vi "AUTON_Index.vi"(0 "Auton Array":dbl[][](array[numeric]), 5 "MeasuredHeading":dbl, 7 "LeftEncoder":dbl, 9 "RightEncoder":dbl) -> (4 "Right Drive":dbl, 6 "Left Drive":dbl, 8 "Harvester":dbl, 10 "Winch":dbl, 14 "Roller":dbl, 15 "Cam":dbl)   [LabVIEW 2013]
uses:
  Robot Global Data.vi
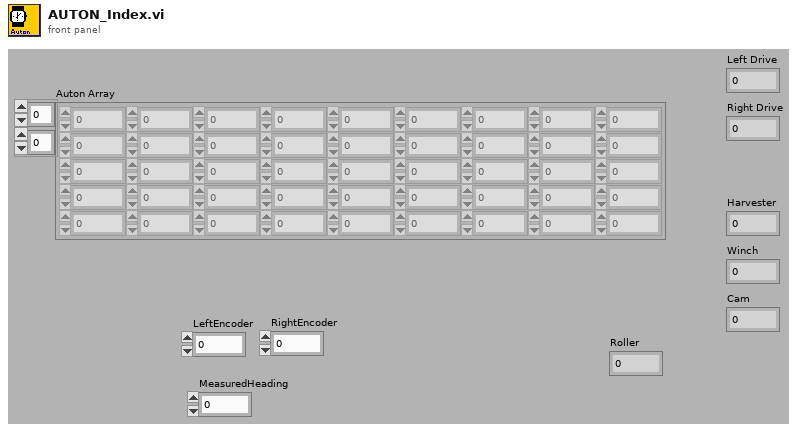
[diagram p1: front panel]
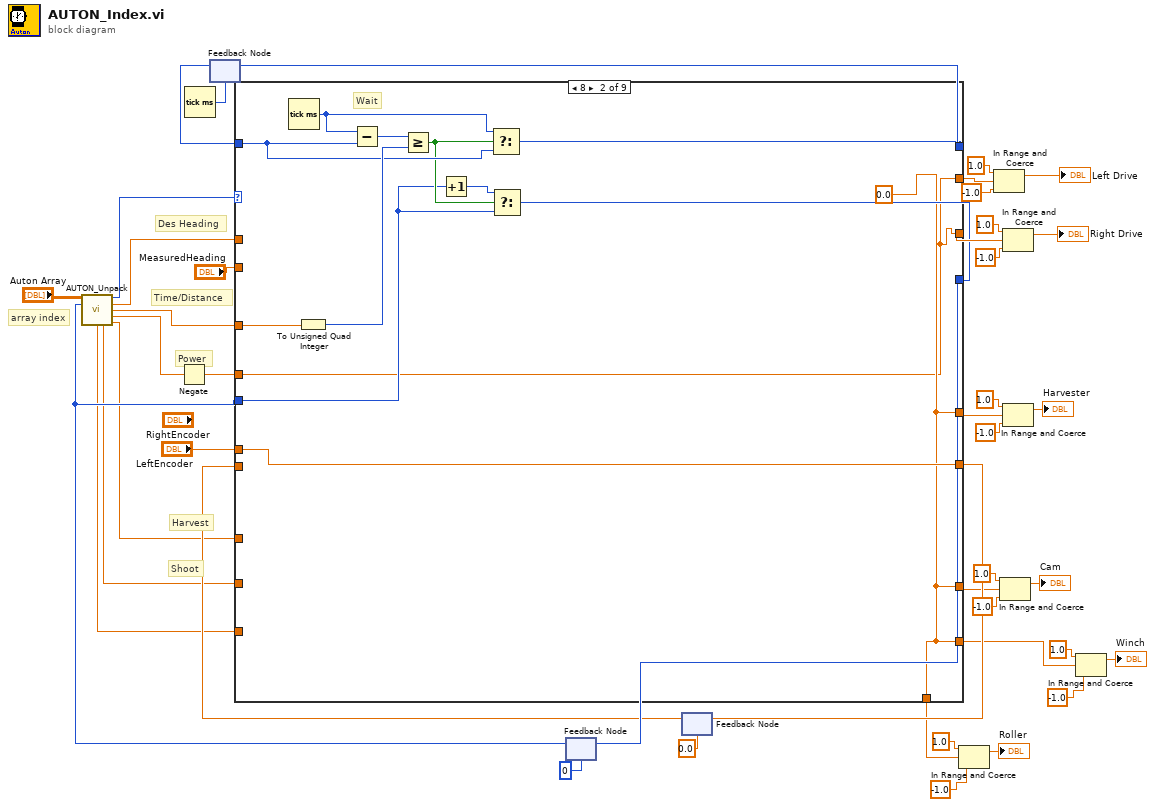
[diagram p0: block diagram]
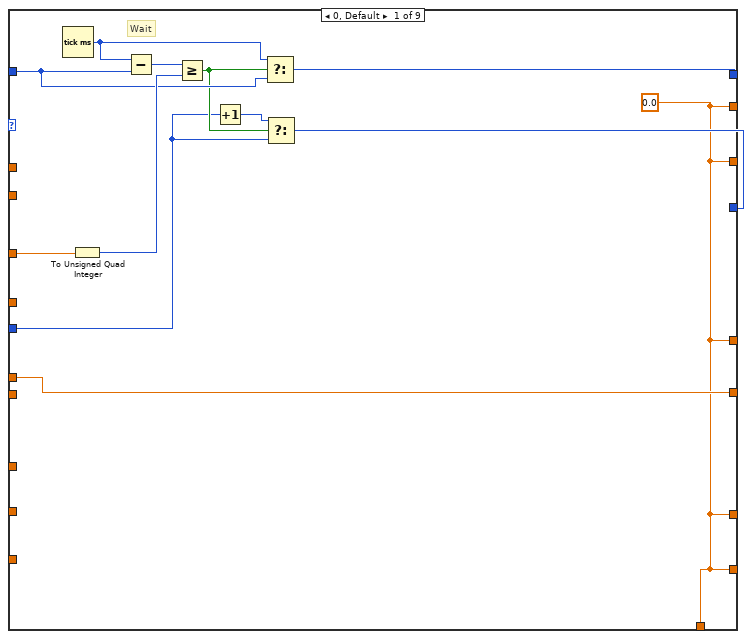
[diagram p2: hidden frame]
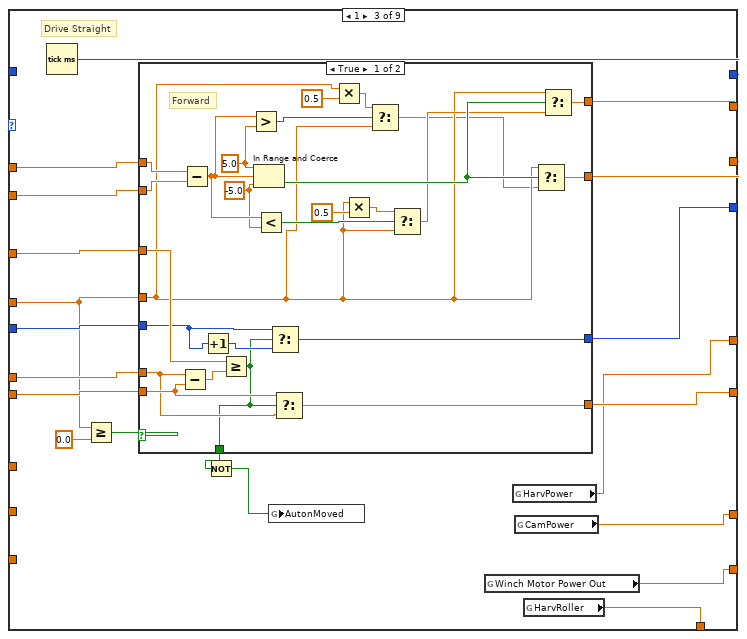
[diagram p3: hidden frame]
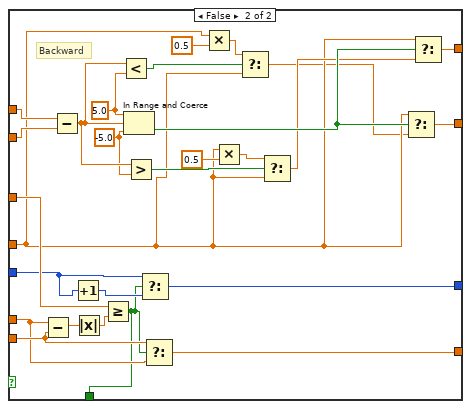
[diagram p4: hidden frame]
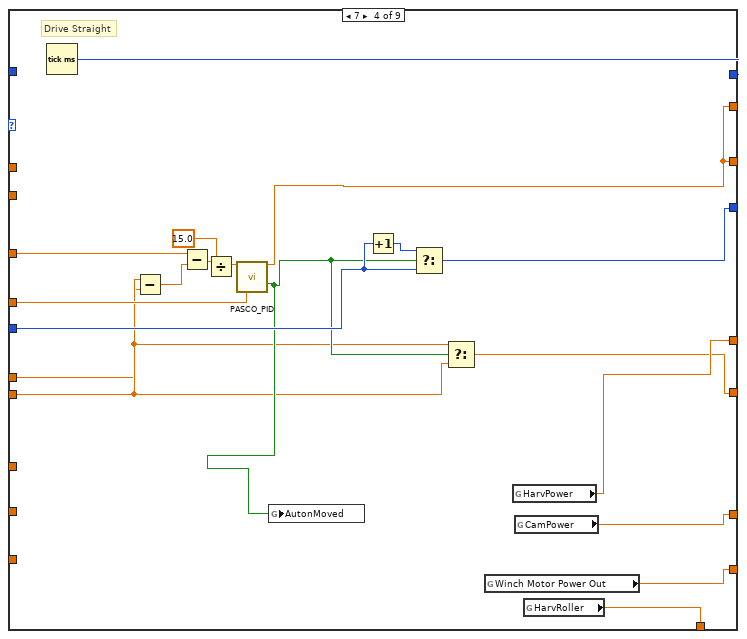
[diagram p5: hidden frame]
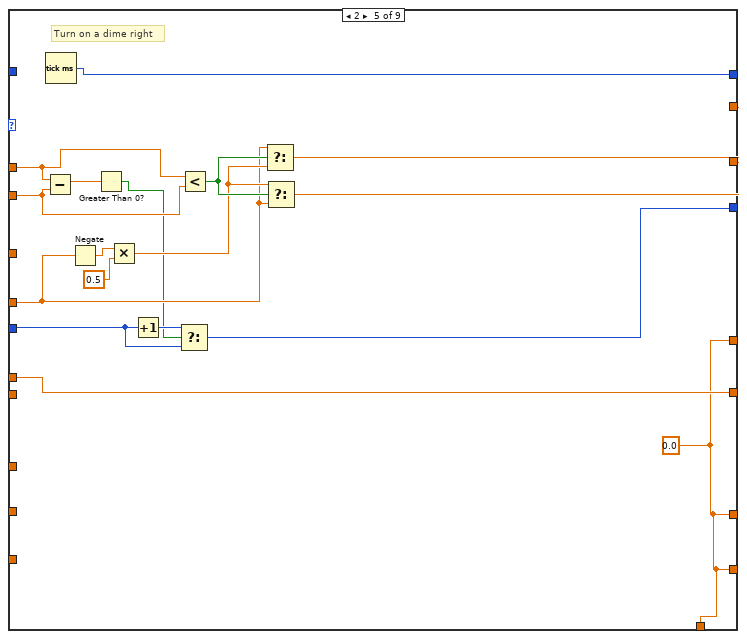
[diagram p6: hidden frame]
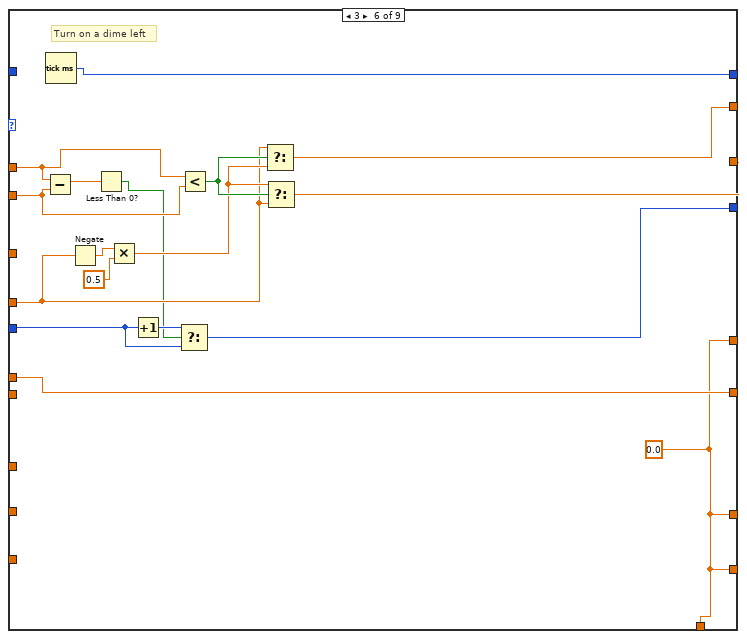
[diagram p7: hidden frame]
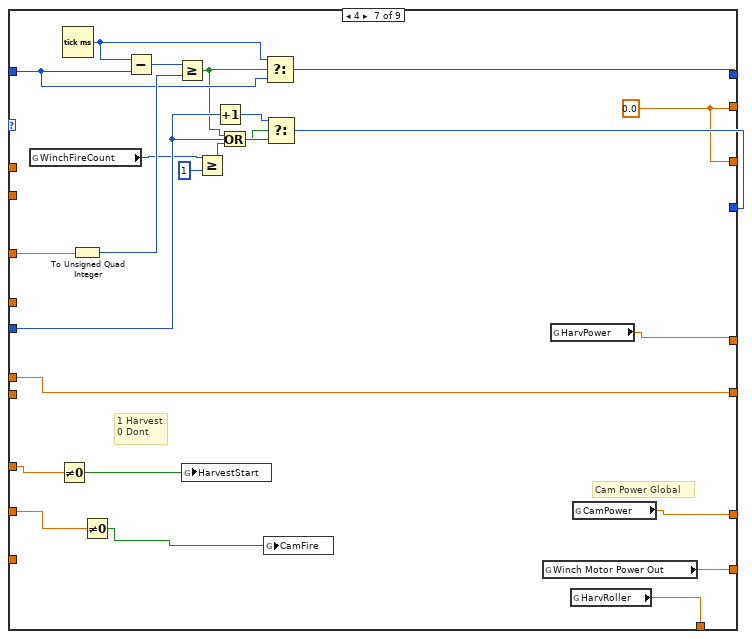
[diagram p8: hidden frame]
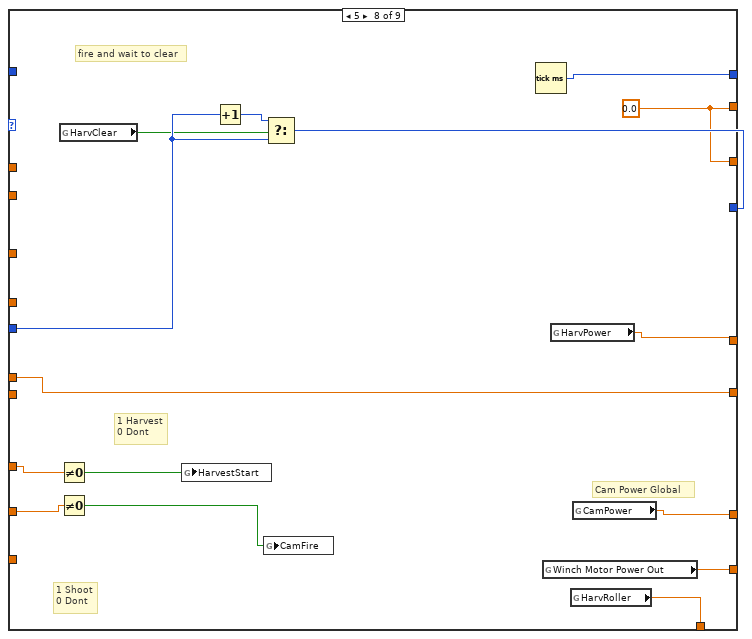
[diagram p9: hidden frame]
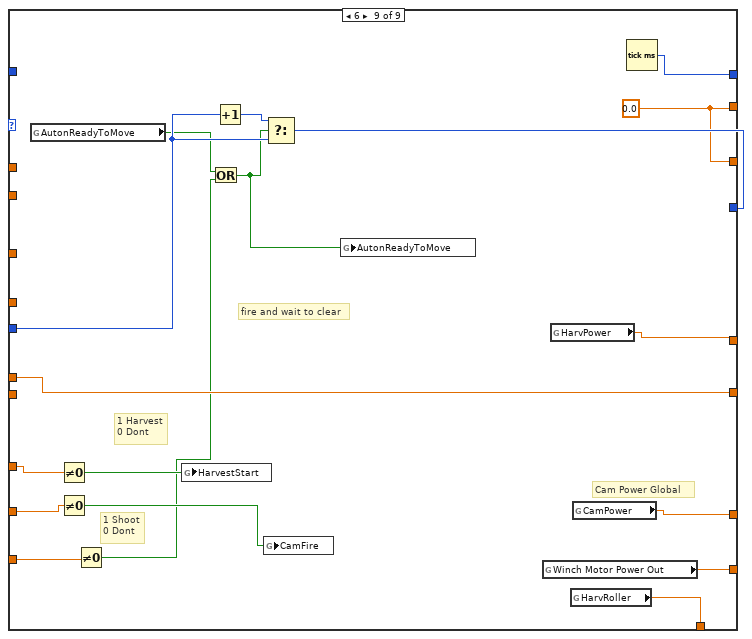
[diagram p10: hidden frame]
diagram:
  # "Shoot"
  # "Harvest"
  # "Des Heading"
  # "Time/Distance"
  # "Power"
  # "array index"
  n1 = Tick Count (ms)() -> (millisecond timer value=w42:u32)
  n2 = feedback #1(w42) -> (w43:u32)
  n3 = feedback #2(0) -> (w23:i32)
  n4 = call "AUTON_Unpack.vi"("all rows"="Auton Array", "Index"=w23) -> ("Primitive ID"=w26:i16, "Desired Heading"=w25:dbl, "Time/Distance"=w24:dbl, "Power"=w11:dbl, "Moved"=w1:dbl, "Shoot"=w8:dbl, "Harvest"=w9:dbl)  [unwired: 7 in]
  n5 = Negate(x=w11) -> (-x=w10:dbl)
  n6 = feedback #3(0.0) -> (w28:dbl)
  n7 = case shown="8" w26 {
    tunnel: [w48 w61 w87 w155 w173 w190 w212 w232 w250] -> w30
    tunnel: w23 -> [w49 w62 w82 w153 w176 w193 w213 w233 w251]
    tunnel: [w56 w69 w79 w161 w178 w195 w219 w223 w239] -> w32
    tunnel: w43 -> [w53 w66 _ _ _ _ w216 _ _]
    tunnel: w24 -> [w47 w60 w88 w145 _ _ w211 _ _]
    tunnel: w25 -> [_ _ w86 _ w171 w188 _ _ _]
    tunnel: [w45 w57 w84 w143 w174 w191 w210 w231 w249] -> w40
    tunnel: [w45 w57 w83 w143 w175 w192 w210 w231 w249] -> w33
    tunnel: w10 -> [_ w57 w78 w156 w165 w182 _ _ _]
    tunnel: "LeftEncoder" -> [w46 w59 w80 w148 w172 w189 w209 w230 w248]
    tunnel: "MeasuredHeading" -> [_ _ w85 _ w170 w187 _ _ _]
    tunnel: w28 -> [_ _ w81 w149 _ _ _ _ _]
    tunnel: [w46 w59 w89 w151 w172 w189 w209 w230 w248] -> w27
    tunnel: [w45 w58 w75 w160 w162 w179 w207 w228 w246] -> w13
    tunnel: [w45 w58 w73 w158 w162 w179 w208 w229 w247] -> w12
    tunnel: w9 -> [_ _ _ _ _ _ w204 w226 w244]
    tunnel: w8 -> [_ _ _ _ _ _ w206 w221 w241]
    tunnel: [w45 w58 w74 w159 w162 w179 w205 w227 w245] -> w7
    tunnel: [w45 w58 w72 w157 w162 w179 w201 w224 w242] -> w3
    tunnel: w1 -> [_ _ _ _ _ _ _ _ w238]
    frame 0, Default {
      w45 = 0.0 ("Numeric")
      # "Wait"
      n8 = Tick Count (ms)() -> (millisecond timer value=w52:u32)
      n9 = To Unsigned Quad Integer(1:w47) -> (0:w54:u64)
      n10 = Subtract(x=w52, y=w53) -> (x-y=w55:u32)
      n11 = Greater Or Equal?(x=w55, y=w54) -> (x >= y?=w51:bool)
      n12 = Increment(x=w49) -> (x+1=w50:i32)
      n13 = Select(t=w52, s=w51, f=w53) -> (s? t:f=w56:u32)
      n14 = Select(t=w50, s=w51, f=w49) -> (s? t:f=w48:i32)
    }
    frame 8 {
      w58 = 0.0 ("Numeric")
      # "Wait"
      n15 = Tick Count (ms)() -> (millisecond timer value=w65:u32)
      n16 = To Unsigned Quad Integer(1:w60) -> (0:w67:u64)
      n17 = Subtract(x=w65, y=w66) -> (x-y=w68:u32)
      n18 = Greater Or Equal?(x=w68, y=w67) -> (x >= y?=w64:bool)
      n19 = Increment(x=w62) -> (x+1=w63:i32)
      n20 = Select(t=w65, s=w64, f=w66) -> (s? t:f=w69:u32)
      n21 = Select(t=w63, s=w64, f=w62) -> (s? t:f=w61:i32)
    }
    frame 1 {
      # "Drive Straight"
      n22 = Tick Count (ms)() -> (millisecond timer value=w79:u32)
      n23 = Greater Or Equal?(x=w78, y=0.0) -> (x >= y?=w76:bool)
      n24 = case shown="True" w76 {
        tunnel: [w115 w142] -> w89
        tunnel: w88 -> [w113 w141]
        tunnel: [w112 w140] -> w87
        tunnel: w86 -> [w111 w139]
        tunnel: w85 -> [w110 w138]
        tunnel: [w108 w136] -> w84
        tunnel: [w107 w135] -> w83
        tunnel: w78 -> [w96 w124]
        tunnel: w82 -> [w93 w121]
        tunnel: w81 -> [w92 w120]
        tunnel: w80 -> [w91 w119]
        tunnel: [w90 w116] -> w71
        frame True {
          w104 = -5.0 ("lower limit")
          w106 = 5.0 ("upper limit")
          # "Forward"
          n25 = Subtract(x=w91, y=w92) -> (x-y=w114:dbl)
          n26 = Subtract(x=w111, y=w110) -> (x-y=w105:dbl)
          n27 = Increment(x=w93) -> (x+1=w94:i32)
          n28 = Greater Or Equal?(x=w113, y=w114) -> (x >= y?=w90:bool)
          n29 = Greater?(x=w105, y=w106) -> (0:w99:bool)
          n30 = In Range and Coerce(upper limit=w106, x=w105, lower limit=w104) -> (In Range?=w109:bool)  [unwired: 1 out]
          n31 = Less?(x=w105, y=w104) -> (x < y?=w103:bool)
          n32 = Select(t=w93, s=w90, f=w94) -> (s? t:f=w112:i32)
          n33 = Select(t=w92, s=w90, f=w91) -> (s? t:f=w115:dbl)
          n34 = Multiply(x=w96, y=0.5) -> (x*y=w98:dbl)
          n35 = Multiply(x=w96, y=0.5) -> (x*y=w101:dbl)
          n36 = Select(t=w98, s=w99, f=w96) -> (s? t:f=w95:dbl)
          n37 = Select(t=w101, s=w103, f=w96) -> (s? t:f=w100:dbl)
          n38 = Select(t=w96, s=w109, f=w95) -> (s? t:f=w107:dbl)
          n39 = Select(t=w96, s=w109, f=w100) -> (s? t:f=w108:dbl)
        }
        frame False {
          w132 = -5.0 ("lower limit")
          w134 = 5.0 ("upper limit")
          # "Backward"
          n40 = Subtract(x=w119, y=w120) -> (x-y=w117:dbl)
          n41 = Subtract(x=w139, y=w138) -> (x-y=w133:dbl)
          n42 = Increment(x=w121) -> (x+1=w122:i32)
          n43 = Absolute Value(x=w117) -> (abs(x)=w118:dbl)
          n44 = Greater Or Equal?(x=w141, y=w118) -> (x >= y?=w116:bool)
          n45 = Less?(x=w133, y=w134) -> (x < y?=w127:bool)
          n46 = In Range and Coerce(upper limit=w134, x=w133, lower limit=w132) -> (In Range?=w137:bool)  [unwired: 1 out]
          n47 = Greater?(x=w133, y=w132) -> (0:w131:bool)
          n48 = Select(t=w121, s=w116, f=w122) -> (s? t:f=w140:i32)
          n49 = Select(t=w120, s=w116, f=w119) -> (s? t:f=w142:dbl)
          n50 = Multiply(x=w124, y=0.5) -> (x*y=w126:dbl)
          n51 = Multiply(x=w124, y=0.5) -> (x*y=w129:dbl)
          n52 = Select(t=w126, s=w127, f=w124) -> (s? t:f=w123:dbl)
          n53 = Select(t=w129, s=w131, f=w124) -> (s? t:f=w128:dbl)
          n54 = Select(t=w124, s=w137, f=w123) -> (s? t:f=w135:dbl)
          n55 = Select(t=w124, s=w137, f=w128) -> (s? t:f=w136:dbl)
        }
      }
      n56 = Not(x=w71) -> (.not. x?=w70:bool)
      n57 = global write "Robot Global Data.vi" "AutonMoved"(w70) -> ()
      n58 = global read "Robot Global Data.vi" "Winch Motor Power Out"() -> (w74:dbl)
      n59 = global read "Robot Global Data.vi" "HarvPower"() -> (w73:dbl)
      n60 = global read "Robot Global Data.vi" "CamPower"() -> (w75:dbl)
      n61 = global read "Robot Global Data.vi" "HarvRoller"() -> (w72:dbl)
    }
    frame 7 {
      # "Drive Straight"
      n62 = Tick Count (ms)() -> (millisecond timer value=w161:u32)
      n63 = Subtract(x=w149, y=w148) -> (x-y=w150:dbl)
      n64 = Subtract(x=w145, y=w150) -> (x-y=w146:dbl)
      n65 = Divide(x=w146, y=15.0) -> (x/y=w147:dbl)
      n66 = call "PASCO_PID.vi"("Delta"=w147, "P Gain"=w156) -> ("Output"=w143:dbl, "IsThere"=w152:bool)  [unwired: 12 in]
      n67 = global write "Robot Global Data.vi" "AutonMoved"(w152) -> ()
      n68 = Increment(x=w153) -> (x+1=w154:i32)
      n69 = Select(t=w154, s=w152, f=w153) -> (s? t:f=w155:i32)
      n70 = Select(t=w148, s=w152, f=w149) -> (s? t:f=w151:dbl)
      n71 = global read "Robot Global Data.vi" "Winch Motor Power Out"() -> (w159:dbl)
      n72 = global read "Robot Global Data.vi" "HarvPower"() -> (w158:dbl)
      n73 = global read "Robot Global Data.vi" "CamPower"() -> (w160:dbl)
      n74 = global read "Robot Global Data.vi" "HarvRoller"() -> (w157:dbl)
    }
    frame 2 {
      w162 = 0.0 ("Numeric")
      # "Turn on a dime right"
      n75 = Subtract(x=w171, y=w170) -> (x-y=w164:dbl)
      n76 = Tick Count (ms)() -> (millisecond timer value=w178:u32)
      n77 = Negate(x=w165) -> (-x=w168:dbl)
      n78 = Greater Than 0?(x=w164) -> (x > 0?=w163:bool)
      n79 = Multiply(x=w168, y=0.5) -> (x*y=w166:dbl)
      n80 = Increment(x=w176) -> (x+1=w177:i32)
      n81 = Select(t=w177, s=w163, f=w176) -> (s? t:f=w173:i32)
      n82 = Less?(x=w171, y=w170) -> (x < y?=w169:bool)
      n83 = Select(t=w165, s=w169, f=w166) -> (s? t:f=w174:dbl)
      n84 = Select(t=w166, s=w169, f=w165) -> (s? t:f=w175:dbl)
    }
    frame 3 {
      w179 = 0.0 ("Numeric")
      # "Turn on a dime left"
      n85 = Subtract(x=w188, y=w187) -> (x-y=w181:dbl)
      n86 = Tick Count (ms)() -> (millisecond timer value=w195:u32)
      n87 = Negate(x=w182) -> (-x=w185:dbl)
      n88 = Less Than 0?(x=w181) -> (x < 0?=w180:bool)
      n89 = Multiply(x=w185, y=0.5) -> (x*y=w183:dbl)
      n90 = Increment(x=w193) -> (x+1=w194:i32)
      n91 = Select(t=w194, s=w180, f=w193) -> (s? t:f=w190:i32)
      n92 = Less?(x=w188, y=w187) -> (x < y?=w186:bool)
      n93 = Select(t=w182, s=w186, f=w183) -> (s? t:f=w191:dbl)
      n94 = Select(t=w183, s=w186, f=w182) -> (s? t:f=w192:dbl)
    }
    frame 4 {
      w210 = 0.0 ("Numeric")
      # "1 Harvest\n0 Dont"
      # "Cam Power Global"
      n95 = global read "Robot Global Data.vi" "WinchFireCount"() -> (w197:i32)
      n96 = Not Equal To 0?(x=w204) -> (x != 0?=w203:bool)
      n97 = Tick Count (ms)() -> (millisecond timer value=w215:u32)
      n98 = To Unsigned Quad Integer(1:w211) -> (0:w217:u64)
      n99 = Not Equal To 0?(x=w206) -> (x != 0?=w202:bool)
      n100 = Subtract(x=w215, y=w216) -> (x-y=w218:u32)
      n101 = Greater Or Equal?(x=w218, y=w217) -> (x >= y?=w199:bool)
      n102 = global write "Robot Global Data.vi" "HarvestStart"(w203) -> ()
      n103 = Greater Or Equal?(x=w197, y=1) -> (x >= y?=w198:bool)
      n104 = Increment(x=w213) -> (x+1=w214:i32)
      n105 = Or(x=w199, y=w198) -> (x .or. y?=w200:bool)
      n106 = global write "Robot Global Data.vi" "CamFire"(w202) -> ()
      n107 = Select(t=w215, s=w199, f=w216) -> (s? t:f=w219:u32)
      n108 = Select(t=w214, s=w200, f=w213) -> (s? t:f=w212:i32)
      n109 = global read "Robot Global Data.vi" "Winch Motor Power Out"() -> (w205:dbl)
      n110 = global read "Robot Global Data.vi" "HarvPower"() -> (w208:dbl)
      n111 = global read "Robot Global Data.vi" "HarvRoller"() -> (w201:dbl)
      n112 = global read "Robot Global Data.vi" "CamPower"() -> (w207:dbl)
    }
    frame 5 {
      w231 = 0.0 ("Numeric")
      # "fire and wait to clear"
      # "1 Harvest\n0 Dont"
      # "1 Shoot\n0 Dont"
      # "Cam Power Global"
      n113 = Not Equal To 0?(x=w226) -> (x != 0?=w225:bool)
      n114 = Not Equal To 0?(x=w221) -> (x != 0?=w220:bool)
      n115 = global read "Robot Global Data.vi" "HarvClear"() -> (w222:bool)
      n116 = global write "Robot Global Data.vi" "HarvestStart"(w225) -> ()
      n117 = Increment(x=w233) -> (x+1=w234:i32)
      n118 = global write "Robot Global Data.vi" "CamFire"(w220) -> ()
      n119 = Select(t=w234, s=w222, f=w233) -> (s? t:f=w232:i32)
      n120 = Tick Count (ms)() -> (millisecond timer value=w223:u32)
      n121 = global read "Robot Global Data.vi" "Winch Motor Power Out"() -> (w227:dbl)
      n122 = global read "Robot Global Data.vi" "HarvPower"() -> (w229:dbl)
      n123 = global read "Robot Global Data.vi" "HarvRoller"() -> (w224:dbl)
      n124 = global read "Robot Global Data.vi" "CamPower"() -> (w228:dbl)
    }
    frame 6 {
      w249 = 0.0 ("Numeric")
      # "fire and wait to clear"
      # "1 Harvest\n0 Dont"
      # "1 Shoot\n0 Dont"
      # "Cam Power Global"
      n125 = global read "Robot Global Data.vi" "AutonReadyToMove"() -> (w236:bool)
      n126 = Not Equal To 0?(x=w244) -> (x != 0?=w243:bool)
      n127 = Not Equal To 0?(x=w241) -> (x != 0?=w240:bool)
      n128 = Not Equal To 0?(x=w238) -> (x != 0?=w237:bool)
      n129 = global write "Robot Global Data.vi" "HarvestStart"(w243) -> ()
      n130 = Or(x=w236, y=w237) -> (x .or. y?=w235:bool)
      n131 = Increment(x=w251) -> (x+1=w252:i32)
      n132 = global write "Robot Global Data.vi" "CamFire"(w240) -> ()
      n133 = Select(t=w252, s=w235, f=w251) -> (s? t:f=w250:i32)
      n134 = global write "Robot Global Data.vi" "AutonReadyToMove"(w235) -> ()
      n135 = global read "Robot Global Data.vi" "Winch Motor Power Out"() -> (w245:dbl)
      n136 = global read "Robot Global Data.vi" "HarvPower"() -> (w247:dbl)
      n137 = global read "Robot Global Data.vi" "HarvRoller"() -> (w242:dbl)
      n138 = global read "Robot Global Data.vi" "CamPower"() -> (w246:dbl)
      n139 = Tick Count (ms)() -> (millisecond timer value=w239:u32)
    }
  }
  n140 = feedback-in #1(w32) -> ()
  n141 = feedback-in #2(w30) -> ()
  n142 = feedback-in #3(w27) -> ()
  n143 = In Range and Coerce(upper limit=1.0, x=w3, lower limit=-1.0) -> (coerced(x)=→"Roller":dbl)  [unwired: 1 out]
  n144 = In Range and Coerce(upper limit=1.0, x=w40, lower limit=-1.0) -> (coerced(x)=→"Left Drive":dbl)  [unwired: 1 out]
  n145 = In Range and Coerce(upper limit=1.0, x=w13, lower limit=-1.0) -> (coerced(x)=→"Cam":dbl)  [unwired: 1 out]
  n146 = In Range and Coerce(upper limit=1.0, x=w33, lower limit=-1.0) -> (coerced(x)=→"Right Drive":dbl)  [unwired: 1 out]
  n147 = In Range and Coerce(upper limit=1.0, x=w12, lower limit=-1.0) -> (coerced(x)=→"Harvester":dbl)  [unwired: 1 out]
  n148 = In Range and Coerce(upper limit=1.0, x=w7, lower limit=-1.0) -> (coerced(x)=→"Winch":dbl)  [unwired: 1 out]
